vi "xxMain_05B.vi"() -> ()   [LabVIEW 2025]
uses:
  Utility/Universal Utility/TypeDefs_Utility/Cluster_Row-Column.ctl
  9e3f57c0-2ef8-4495-8287-c6a42a5fb955.vi
  Utility/Universal Utility/TypeDefs_Utility/ENUM_4 Directions U-D-L-R.ctl
  Utility/Universal Utility/TypeDefs_Utility/ENUM_8 Directions U-D-L-R.ctl
panel:
  out "Min":u64[](array[numeric])
  out "max":u64[](array[numeric])
  out "x-1":u64
  out "MATCH":bool
  in  "Select Data":enum32{"Example", "Puzzle"}(tab)
  in  "EX Target":u32=14
  in  "Example":string="3-5\n10-14\n16-20\n12-18\n\n1\n5\n8\n11\n17\n32"
  in  "Puzzle":string="505104443555011-505832008521290\n183705568221799-189071596736306\n25714421842394-26498060657296\n324591982604436-326326266144576\n194954655268286-199771011784310\n32539515377401-39552166142220\n326326266144577-330576407995732\n45877724695638-45877724695638\n245990755269494-248893742631986\n316826876448244-321016747706186\n23726069480801-24221552311396\n282687875186245-282687875186245\n84944235636755-86138442862850\n27463398169403-27981167005022\n388889831860114-389071080230049\n178876097666360-180498038018267\n509753176570993-510393291709325\n137682268842164-139478866740539\n504458187396917-505104443555011\n5030..."
  in  "Puzzle Target":u32
  out "Answer":u64
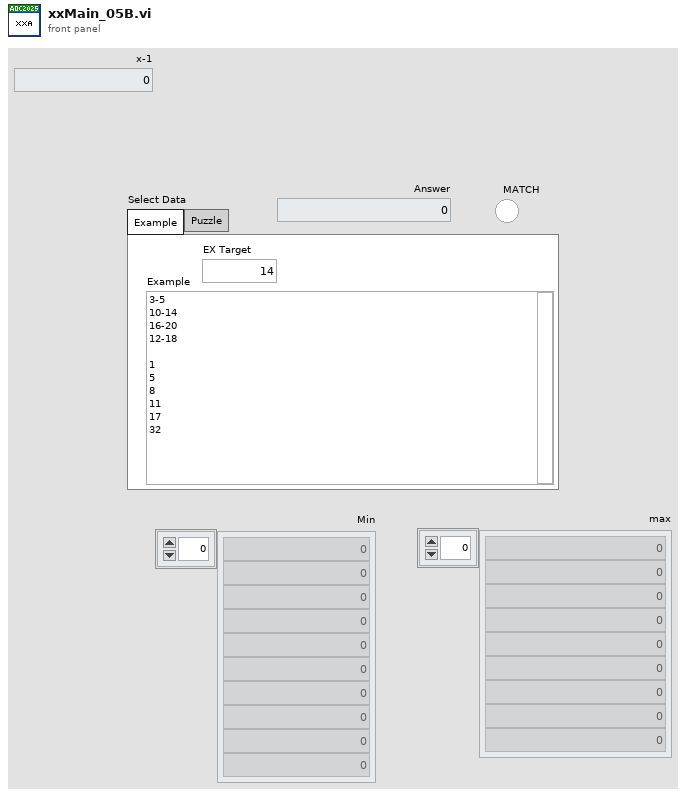
[diagram p1: front panel]
types:
  T1 = typedef "ENUM_8 Directions U-D-L-R.ctl" = enum16{"Up;-1,0", "Up-Right;-1,1", "Right;0,1", "Down-Right;1,1", "Down;1,0", "Down-Left;1,-1", "Left;0,-1", "Up-Left;-1,-1"}
  T2 = typedef "ENUM_4 Directions U-D-L-R.ctl" = enum16{"Up;-1,0", "Right;0,1", "Down;1,0", "Left;0,-1"}
  T3 = typedef "Cluster_Row-Column.ctl" = cluster{"R":i32, "C":i32}
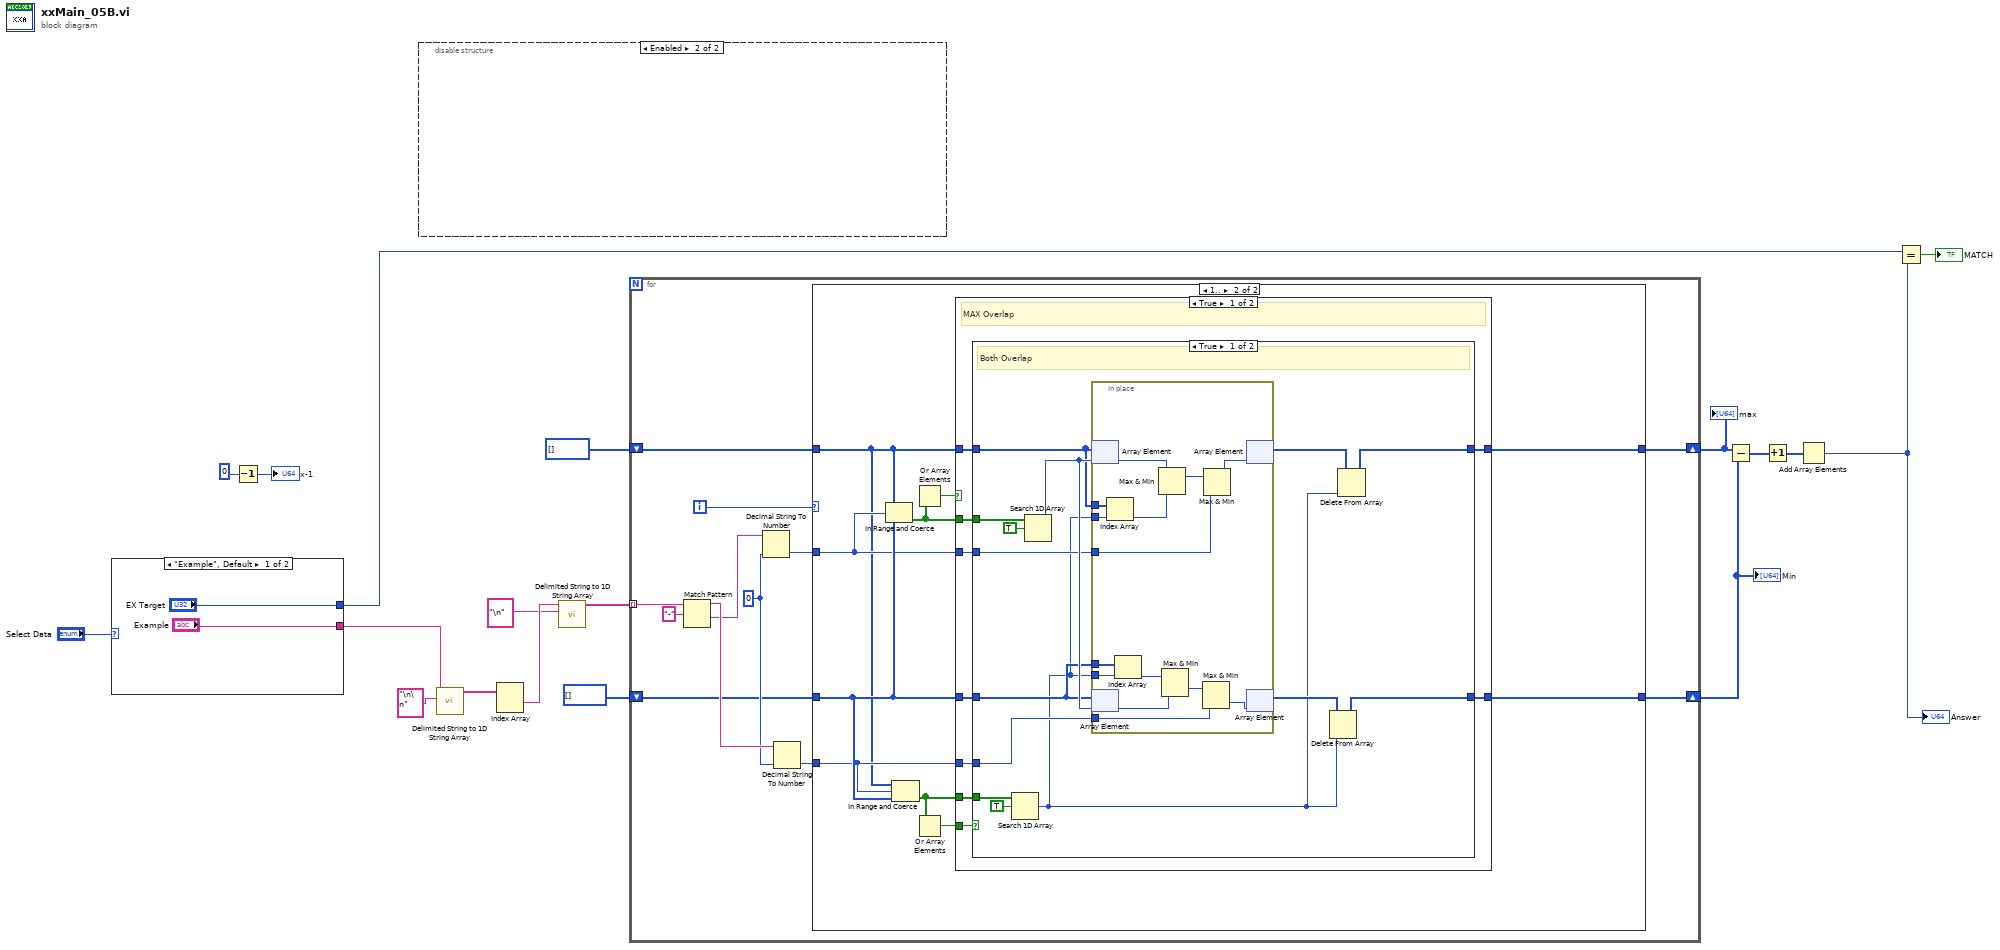
[diagram p0: block diagram]
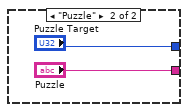
[diagram p2: hidden frame]
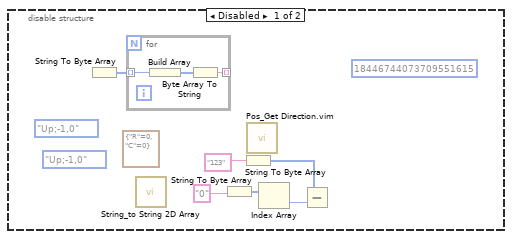
[diagram p3: hidden frame]
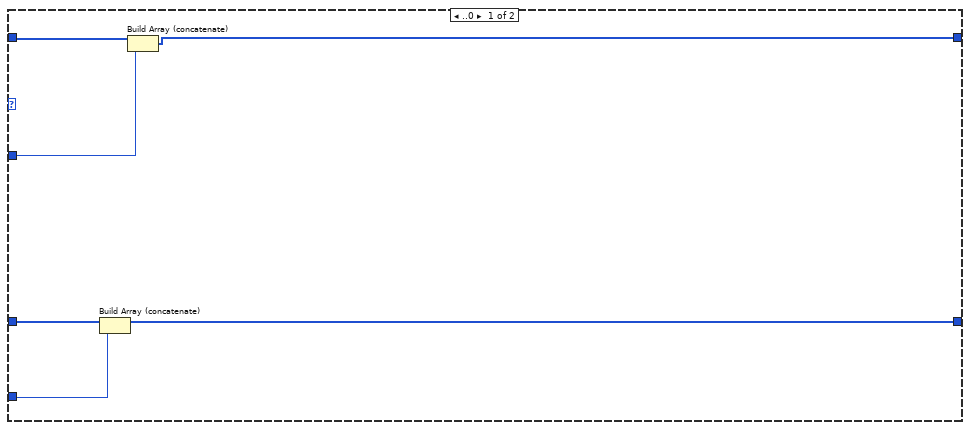
[diagram p4: hidden frame]
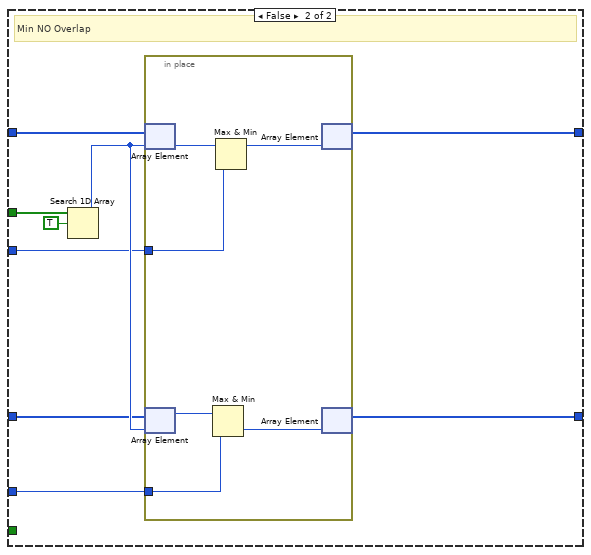
[diagram p5: hidden frame]
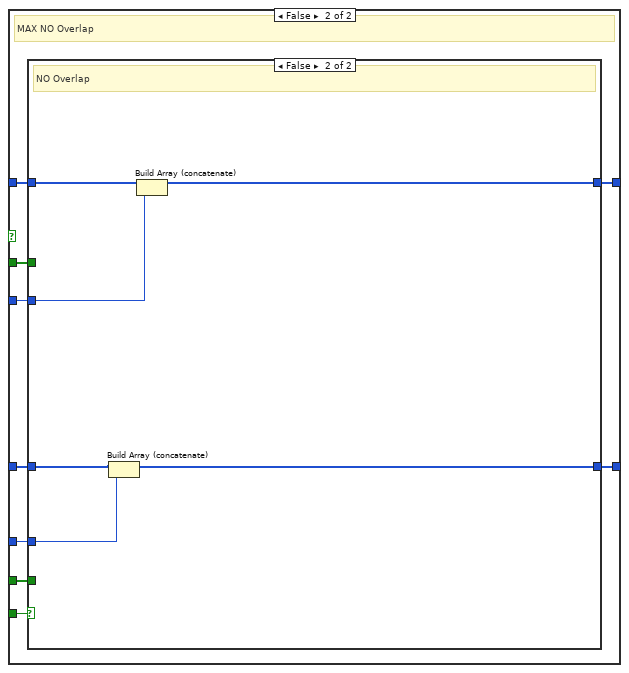
[diagram p6: hidden frame]
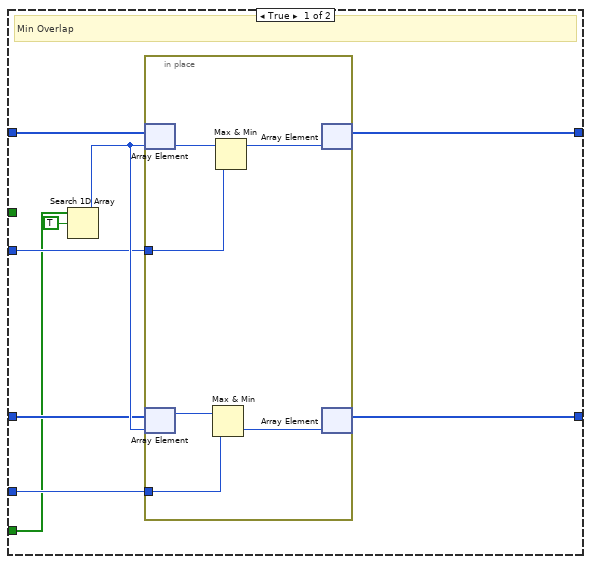
[diagram p7: hidden frame]
diagram:
  n1 = case shown="\"Example\", Default" "Select Data" {
    tunnel: ["Example" "Puzzle"] -> w17
    tunnel: ["EX Target" "Puzzle Target"] -> w14
    frame "Example", Default {
    }
    frame "Puzzle" {
    }
  }
  n2 = Decrement(x=u64 0) -> (x-1=→"x-1":u64)
  n3 = disable-structure shown="Enabled" {
    frame Disabled {
      (unwired) u64 18446744073709551615 ("x-1")
      (unwired) ENUM_8_Directions_U-D-L-R."Up;-1,0" ("Direction 8")
      (unwired) ENUM_4_Directions_U-D-L-R."Up;-1,0" ("Direction")
      (unwired) T3 {"R"=0, "C"=0} ("Position")
      n4 = String To Byte Array() -> (unsigned byte array=w23:u8[])  [unwired: 1 in]
      n5 = for {
        tunnel: w23 -> [w31] mode=indexing
        tunnel: [w29] -> _ mode=indexing
        n6 = Build Array(w31) -> (w30:u8[])
        n7 = Byte Array To String(unsigned byte array=w30) -> (string=w29:string)
      }
      n8 = call "String_to String 2D Array.vi"() -> ()  [unwired: 11 in, 1 out]
      n9 = String To Byte Array(string="0") -> (unsigned byte array=w26:u8[])
      n10 = String To Byte Array(string="123") -> (unsigned byte array=w24:u8[])
      n11 = call "Pos_Get Direction.vim"() -> ()  [unwired: 11 in, 1 out]
      n12 = Index Array(array=w26) -> (element=w25:u8)  [unwired: 1 in]
      n13 = Subtract(x=w24, y=w25) -> ()  [unwired: 1 out]
    }
    frame Enabled {
    }
  }
  n14 = call <vilib>:"Delimited String to 1D String Array.vi"("delimiter"="\n\n" ("delimiter (Tab)"), "delimited string"=w17) -> ("string array"=w11:string[])  [unwired: 9 in]
  n15 = Index Array(array=w11) -> (element #1=w10:string)  [unwired: 2 in, 1 out]
  n16 = call <vilib>:"Delimited String to 1D String Array.vi"("delimiter"="\n" ("delimiter (Tab)"), "delimited string"=w10) -> ("string array"=w8:string[])  [unwired: 9 in]
  n17 = for {
    tunnel: w8 -> [w43] mode=indexing
    shift-right: [w32] -> w5
    shift-left: u64[] [] ("default (0 I32)") -> [w37]
    shift-right: [w33] -> w4
    shift-left: u64[] [] ("default (0 I32)") -> [w36]
    i -> [w38]
    w39 = u64 0 ("default (0 I32)")
    n18 = Match Pattern(string=w43, regular expression="-") -> (before substring=w41:string, after substring=w40:string)  [unwired: 1 in, 2 out]
    n19 = Decimal String To Number(string=w40, default (0L)=w39) -> (number=w35:u64)  [unwired: 1 in, 1 out]
    n20 = Decimal String To Number(string=w41, default (0L)=w39) -> (number=w34:u64)  [unwired: 1 in, 1 out]
    n21 = case shown="1.." w38 {
      tunnel: w37 -> [w49 w52]
      tunnel: w36 -> [w47 w55]
      tunnel: w35 -> [w48 w53]
      tunnel: w34 -> [w46 w54]
      tunnel: [w45 w51] -> w33
      tunnel: [w44 w50] -> w32
      frame ..0 {
        n22 = Build Array (concatenate)(w47, w46) -> (w45:u64[])
        n23 = Build Array (concatenate)(w49, w48) -> (w44:u64[])
      }
      frame 1.. {
        n24 = In Range and Coerce(upper limit=w52, x=w53, lower limit=w55) -> (In Range?=w57:bool[])  [unwired: 1 out]
        n25 = In Range and Coerce(upper limit=w52, x=w54, lower limit=w55) -> (In Range?=w56:bool[])  [unwired: 1 out]
        n26 = Or Array Elements(Boolean array=w57) -> (logical OR=w59:bool)
        n27 = Or Array Elements(Boolean array=w56) -> (logical OR=w58:bool)
        n28 = case shown="True" w59 {
          tunnel: w58 -> [w68 w120]
          tunnel: w57 -> [w67 w119]
          tunnel: w56 -> [w66 w118]
          tunnel: w55 -> [w65 w117]
          tunnel: w54 -> [w64 w116]
          tunnel: w53 -> [w63 w115]
          tunnel: w52 -> [w62 w114]
          tunnel: [w61 w113] -> w51
          tunnel: [w60 w112] -> w50
          frame True {
            # "MAX Overlap"
            n29 = case shown="True" w68 {
              tunnel: w67 -> [w82 w105]
              tunnel: w66 -> [w80 _]
              tunnel: w65 -> [w76 w101]
              tunnel: w64 -> [w74 w99]
              tunnel: w63 -> [w75 w100]
              tunnel: w62 -> [w77 w102]
              tunnel: [w72 w97] -> w61
              tunnel: [w70 w98] -> w60
              frame True {
                # "Both Overlap"
                n30 = Search 1D Array(1D array=w80, element=TRUE) -> (index of element=w69:i32)  [unwired: 1 in]
                n31 = Search 1D Array(1D array=w82, element=TRUE) -> (index of element=w78:i32)  [unwired: 1 in]
                n32 = in-place {
                  in-place-border: w77 -> [w96]
                  in-place-border: w76 -> [w95]
                  in-place-border: w69 -> [w94]
                  in-place-border: w69 -> [w93]
                  in-place-border: w75 -> [w90]
                  in-place-border: w74 -> [w84]
                  n33 = in-place-array #1(w77, w78) -> (w92:u64)
                  n34 = in-place-array #2(w76, w78) -> (w86:u64)
                  n35 = Index Array(array=w96, index=w93) -> (element=w91:u64)
                  n36 = Index Array(array=w95, index=w94) -> (element=w87:u64)
                  n37 = Max & Min(x=w92, y=w91) -> (max(x,y)=w89:u64)  [unwired: 1 out]
                  n38 = Max & Min(x=w87, y=w86) -> (min(x,y)=w85:u64)  [unwired: 1 out]
                  n39 = Max & Min(x=w85, y=w84) -> (min(x,y)=w83:u64)  [unwired: 1 out]
                  n40 = Max & Min(x=w89, y=w90) -> (max(x,y)=w88:u64)  [unwired: 1 out]
                  n41 = in-place-array #1(w88) -> (w71:u64[])  [unwired: 1 out]
                  n42 = in-place-array #2(w83) -> (w73:u64[])  [unwired: 1 out]
                }
                n43 = Delete From Array(array=w73, index=w69) -> (array with subset deleted=w72:u64[])  [unwired: 1 in, 1 out]
                n44 = Delete From Array(array=w71, index=w69) -> (array with subset deleted=w70:u64[])  [unwired: 1 in, 1 out]
              }
              frame False {
                # "Min NO Overlap"
                n45 = Search 1D Array(1D array=w105, element=TRUE) -> (index of element=w103:i32)  [unwired: 1 in]
                n46 = in-place {
                  in-place-border: w100 -> [w111]
                  in-place-border: w99 -> [w109]
                  n47 = in-place-array #3(w102, w103) -> (w107:u64)
                  n48 = in-place-array #4(w101, w103) -> (w106:u64)
                  n49 = Max & Min(x=w106, y=w109) -> (min(x,y)=w108:u64)  [unwired: 1 out]
                  n50 = Max & Min(x=w107, y=w111) -> (max(x,y)=w110:u64)  [unwired: 1 out]
                  n51 = in-place-array #3(w110) -> (w98:u64[])  [unwired: 1 out]
                  n52 = in-place-array #4(w108) -> (w97:u64[])  [unwired: 1 out]
                }
              }
            }
          }
          frame False {
            # "MAX NO Overlap"
            n53 = case shown="False" w120 {
              tunnel: w119 -> [_ _]
              tunnel: w118 -> [w121 _]
              tunnel: w117 -> [w126 w139]
              tunnel: w116 -> [w124 w138]
              tunnel: w115 -> [w125 w140]
              tunnel: w114 -> [w127 w141]
              tunnel: [w122 w137] -> w113
              tunnel: [w123 w136] -> w112
              frame True {
                # "Min Overlap"
                n54 = Search 1D Array(1D array=w121, element=TRUE) -> (index of element=w128:i32)  [unwired: 1 in]
                n55 = in-place {
                  in-place-border: w125 -> [w135]
                  in-place-border: w124 -> [w133]
                  n56 = in-place-array #5(w127, w128) -> (w131:u64)
                  n57 = in-place-array #6(w126, w128) -> (w130:u64)
                  n58 = Max & Min(x=w130, y=w133) -> (min(x,y)=w132:u64)  [unwired: 1 out]
                  n59 = Max & Min(x=w131, y=w135) -> (max(x,y)=w134:u64)  [unwired: 1 out]
                  n60 = in-place-array #5(w134) -> (w123:u64[])  [unwired: 1 out]
                  n61 = in-place-array #6(w132) -> (w122:u64[])  [unwired: 1 out]
                }
              }
              frame False {
                # "NO Overlap"
                n62 = Build Array (concatenate)(w139, w138) -> (w137:u64[])
                n63 = Build Array (concatenate)(w141, w140) -> (w136:u64[])
              }
            }
          }
        }
      }
    }
  }
  "max" <- w5
  "Min" <- w4
  n64 = Subtract(x=w5, y=w4) -> (x-y=w3:u64[])
  n65 = Increment(x=w3) -> (x+1=w2:u64[])
  n66 = Add Array Elements(numeric array=w2) -> (sum=w1:u64)
  "Answer" <- w1
  n67 = Equal?(x=w14, y=w1) -> (x = y?=→"MATCH":bool)
